vi "Read Refresh Timeout (ms).vi"(8 "error in (no error)":errorcluster, 11 "UI Window in":refnum<class "UI Window.lvclass">) -> (0 "error out":errorcluster, 2 "Refresh Timeout (ms)":i32=100, 3 "UI Window out":refnum<class "UI Window.lvclass">)   [LabVIEW 2015, in "UI Window.lvlib" / "UI Window.lvclass"]
uses:
  UI Window.lvclass
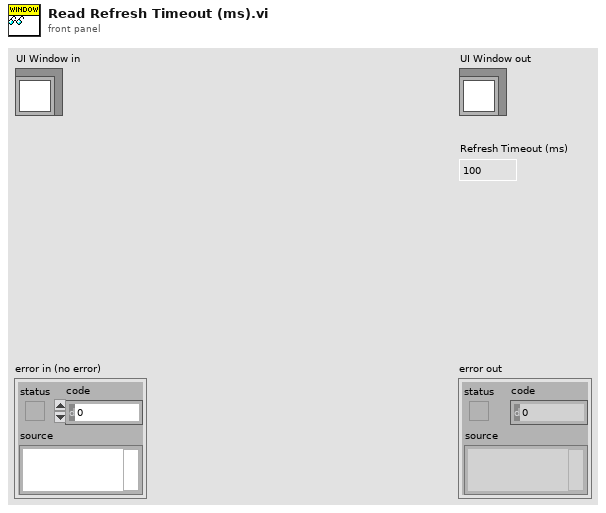
[diagram p1: front panel]
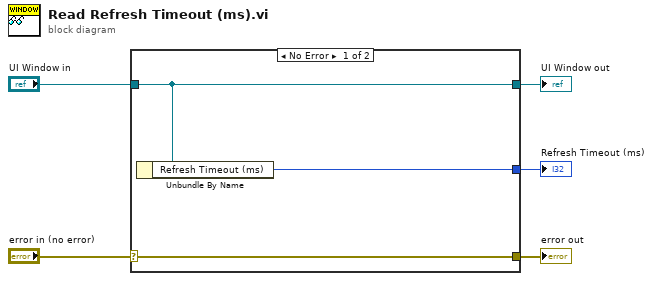
[diagram p0: block diagram]
diagram:
  n1 = case shown="No Error" "error in (no error)" {
    selector: "error in (no error)" -> [w8 w9]
    tunnel: [w8 w9] -> w4
    tunnel: [w7 w10] -> w2
    tunnel: "UI Window in" -> [w7 w10]
    tunnel: [w6 _] -> w1
    frame No Error {
      n2 = Unbundle By Name(w7) -> ("Refresh Timeout (ms)"=w6:i32)
    }
    frame Error {
    }
  }
  "error out" <- w4
  "UI Window out" <- w2
  "Refresh Timeout (ms)" <- w1
